vi "CRYSet Listbox Front Panel.vi"(11 "Vi Ref":refnum<vi>) -> ()   [LabVIEW 2013]
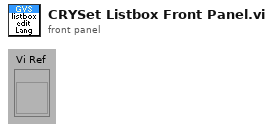
[diagram p1: front panel]
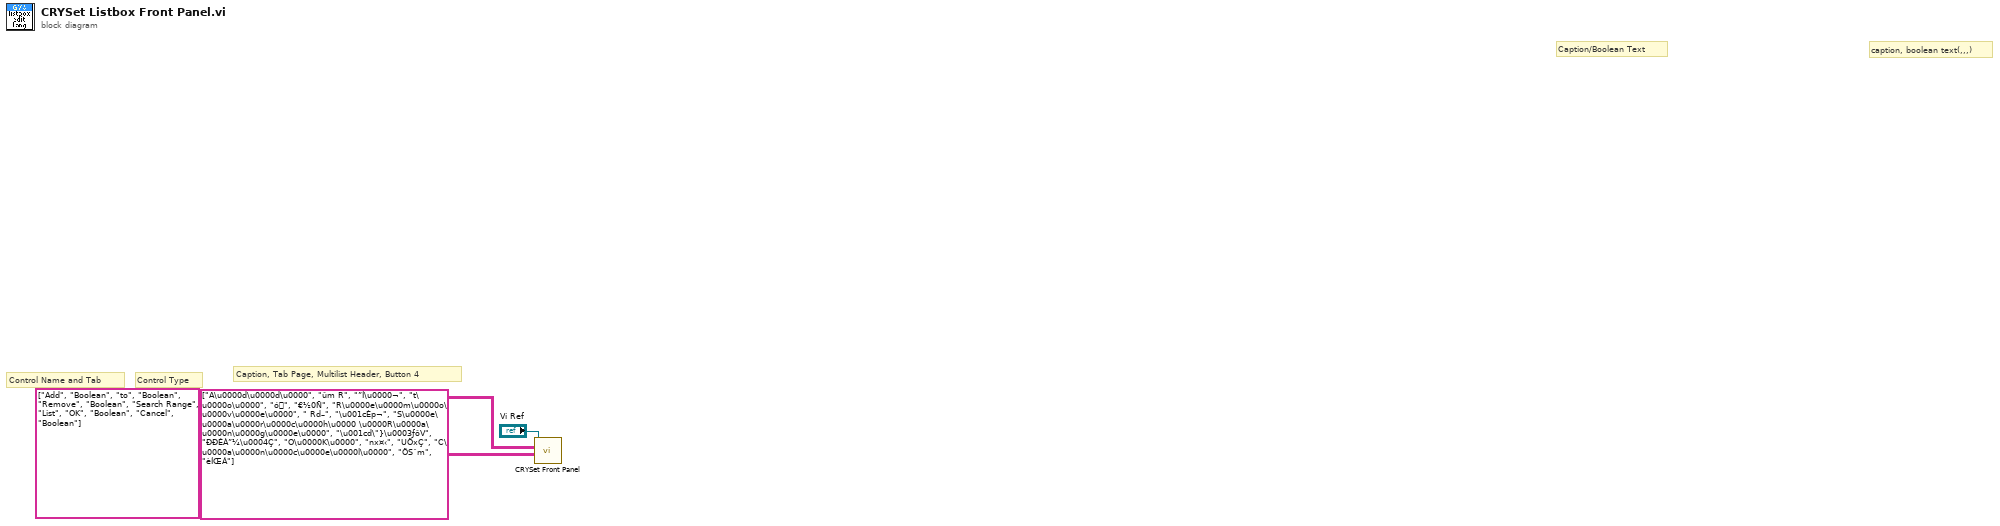
[diagram p0: block diagram]
diagram:
  # "Caption, Tab Page, Multilist Header, Button 4"
  # "Control Type"
  # "Control Name and Tab"
  # "caption, boolean text(,,,)"
  # "Caption/Boolean Text"
  n1 = call "CRYSet Front Panel.vi"("Caption(Boolean Text)"=string[][] [["A\u0000d\u0000d\u0000", "ûm R", "”Í\u0000¬"], ["t\u0000o\u0000", "ó", "€½0Ñ"], ["R\u0000e\u0000m\u0000o\u0000v\u0000e\u0000", " Rd–", "\u001cÈp¬"], ["S\u0000e\u0000a\u0000r\u0000c\u0000h\u0000 \u0000R\u0000a\u0000n\u0000g\u0000e\u0000", "\u001cd\"}\u0003ƒôV", "ÐÐÉÀ”¼\u0004Ç"], ["O\u0000K\u0000", "nx¤‹", "UÖxÇ"], ["C\u0000a\u0000n\u0000c\u0000e\u0000l\u0000", "ÖSˆm", "èÍŒÁ"]], "Control ID and Type(Label Name, Type)"=string[][] [["Add", "Boolean"], ["to", "Boolean"], ["Remove", "Boolean"], ["Search Range", "List"], ["OK", "Boolean"], ["Cancel", "Boolean"]], "Vi Ref"="Vi Ref") -> ()  [unwired: 9 in]
